vi "Plane.ReftoDVR.vi"(10 "Ref":u32 format="%08x") -> (2 "Ref":T1)   [LabVIEW 2020, in "Plane.lvclass"]
doc: "JKI State Machine Objects (SMO) 1.0.0.5\nJKI - JKI\nCopyright (c) 2016, JKI"
uses:
  Plane.lvclass
  Typedefs/PrivateData--Ref.ctl
  Typedefs/PrivateData--Cluster.ctl
  Typedefs/Configuration--Cluster.ctl
  Typedefs/PublicEvents--Cluster.ctl
  Typedefs/DataChanged--EventData--Cluster.ctl
  Typedefs/ProtectedEvents--Cluster.ctl
  Typedefs/API Inputs--Cluster.ctl
  Plane.lvclass/Plane.ctl
  Typedefs/PrivateEvents--Cluster.ctl
  Typedefs/PrivateEvents--Plane.SetLatitude.ctl
  Typedefs/PrivateEvents--Plane.SetLongitude.ctl
  Typedefs/PrivateEvents--Plane.SetCoord.ctl
  Typedefs/PrivateEvents--Plane.SetAltitude.ctl
  Typedefs/PrivateEvents--Plane.SetHeading.ctl
  Typedefs/PrivateEvents--Plane.SetSpeed.ctl
  Typedefs/PrivateEvents--Plane.SetICAO.ctl
  Typedefs/PrivateEvents--Plane.SetHDG.ctl
  Typedefs/PrivateEvents--Plane.GetPlaneData.ctl
  Typedefs/PrivateEvents--Plane.SetUpdateTime.ctl
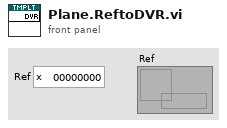
[diagram p1: front panel]
types:
  T1 = typedef "Plane.lvclass/PrivateData--Ref.ctl" = refnum<data-value>
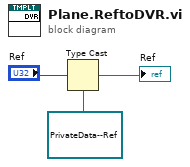
[diagram p0: block diagram]
diagram:
  n1 = Type Cast(type=T1 refnum ("Ref"), x="Ref") -> (*(type *) &x=→"Ref":T1)
